vi "OpenFile.vi"(0 "object in":refnum<class "ErrorLogFile.lvclass">, 2 "Name":string, 5 "Error In":errorcluster) -> (14 "object out":refnum<class "ErrorLogFile.lvclass">, 19 "Error Out":errorcluster)   [LabVIEW 2019, in "ErrorLogFile.lvclass"]
uses:
  ErrorLogFile.lvclass
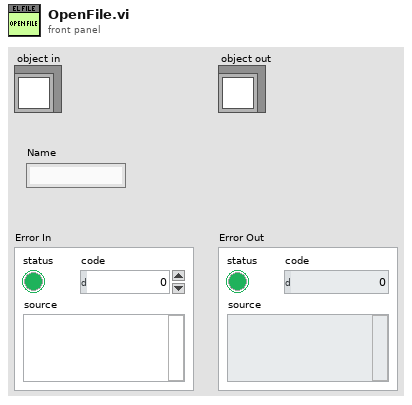
[diagram p1: front panel]
types:
  T1 = enum16{"open", "replace", "create", "open or create", "replace or create", "replace or create with confirmation"}
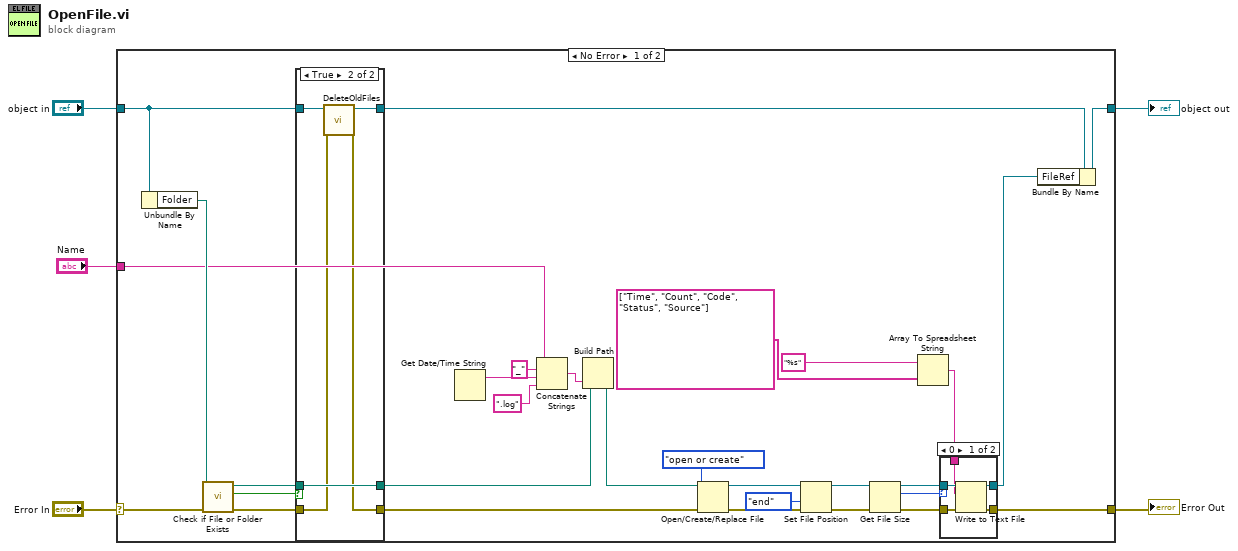
[diagram p0: block diagram]
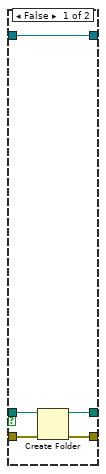
[diagram p3: hidden frame]
diagram:
  n1 = case shown="No Error" "Error In" {
    selector: "Error In" -> [w14 w54]
    tunnel: [w13 w54] -> w4
    tunnel: [w11 w53] -> w2
    tunnel: "object in" -> [w9 w53]
    tunnel: "Name" -> [w6 _]
    frame No Error {
      n2 = Unbundle By Name(w9) -> ("Folder"=w12:path)
      n3 = call <vilib>:"Check if File or Folder Exists.vi"("error in (no error)"=w14, "path"=w12) -> ("error out"=w31:errorcluster, "file or folder exists?"=w27:bool, "dup path"=w28:path)  [unwired: 7 in]
      n4 = case shown="True" w27 {
        tunnel: w31 -> [w47 w50]
        tunnel: [w46 w51] -> w30
        tunnel: [w45 w52] -> w25
        tunnel: w28 -> [w44 w52]
        tunnel: w9 -> [w43 w49]
        tunnel: [w43 w48] -> w8
        frame False {
          n5 = Create Folder(path (use dialog)=w44, error in=w47) -> (created path=w45:path, error out=w46:errorcluster)  [unwired: 1 in, 1 out]
        }
        frame True {
          n6 = call "DeleteOldFiles.vi"("object in"=w49, "Error In"=w50) -> ("object out"=w48:refnum<class "ErrorLogFile.lvclass">, "Error Out"=w51:errorcluster)  [unwired: 16 in]
        }
      }
      n7 = Get Date/Time String() -> (date string=w24:string)  [unwired: 3 in, 1 out]
      n8 = Concatenate Strings(w6, "_" ("string"), w24, ".log" ("string")) -> (w23:string)
      n9 = Build Path(base path=w25, name or relative path=w23) -> (appended path=w26:path)
      n10 = Open/Create/Replace File(file path (use dialog)=w26, error in=w30, operation (0:open)=T1."open or create") -> (refnum out=w33:refnum<file>, error out=w35:errorcluster)  [unwired: 3 in, 1 out]
      n11 = Set File Position(refnum=w33, from (0:start)=enum16{"start", "end", "current"}."end", error in=w35) -> (refnum out=w17:refnum<file>, error out=w29:errorcluster)  [unwired: 1 in]
      n12 = Get File Size(file=w17, error in=w29) -> (refnum out=w16:refnum<file>, size (in bytes)=w15:i64, 0:w18:errorcluster)
      n13 = Array To Spreadsheet String(array=string[] ["Time", "Count", "Code", "Status", "Source"] ("text"), 3:"%s" ("format string")) -> (spreadsheet string=w20:string)  [unwired: 1 in]
      n14 = case shown="0" w15 {
        tunnel: w18 -> [w40 w42]
        tunnel: [w39 w42] -> w13
        tunnel: w16 -> [w38 w41]
        tunnel: [w37 w41] -> w10
        tunnel: w20 -> [w36 _]
        frame 0 {
          n15 = Write to Text File(file (use dialog)=w38, text=w36, error in=w40) -> (refnum out=w37:refnum<file>, error out=w39:errorcluster)  [unwired: 1 in, 1 out]
        }
        frame Default {
        }
      }
      n16 = Bundle By Name(cluster=w8, "FileRef"=w10) -> (w11:refnum<class "ErrorLogFile.lvclass">)
    }
    frame Error {
    }
  }
  "Error Out" <- w4
  "object out" <- w2
